vi "Clear.vi"(8 "error in (no error)":errorcluster, 11 "Engine Simulation Session":refnum<class "Engine Simulation Session.lvclass">) -> (0 "error out":errorcluster)   [LabVIEW 2013, in "Engine Simulation Session.lvclass"]
uses:
  Engine Simulation Session.lvclass
  Engine Simulation Session.lvclass/Engine Simulation Session.ctl
  <vilib>/FPGAPlugInAG/Dynamic/niLvFpga_Close_Dynamic.vi
  <vilib>/rvi/interface/nirviCloseFPGA/nirviCloseFPGA.xnode
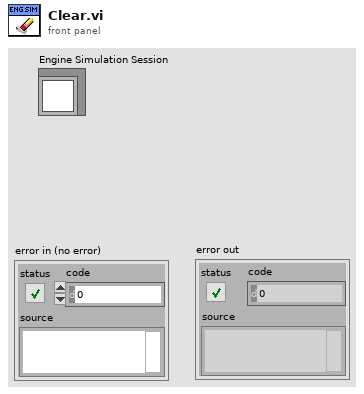
[diagram p1: front panel]
types:
  T1 = typedef "Engine Simulation Session.lvclass/session class private data.ctl" = cluster{"running":bool, "fpga reference":refnum<k20>, "bitfile":path}
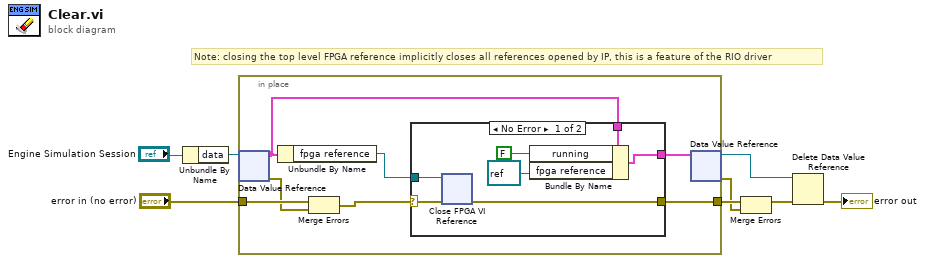
[diagram p0: block diagram]
diagram:
  # "Note: closing the top level FPGA reference implicitly closes all references opened by IP, this is a feature of the RIO driver"
  n1 = Unbundle By Name("Engine Simulation Session") -> ("data"=w7:refnum<data-value>)
  n2 = in-place {
    in-place-border: "error in (no error)" -> [w13]
    in-place-border: [w11] -> w5
    n3 = in-place-dvr #1(w7) -> (w15:T1, w10:errorcluster)
    n4 = Unbundle By Name(w15) -> ("fpga reference"=w12:refnum<k20>)
    n5 = Merge Errors(w13, w10) -> (w9:errorcluster)
    n6 = case shown="No Error" w9 {
      selector: w9 -> [w16 w23]
      tunnel: w15 -> [w22 w24]
      tunnel: [w20 w24] -> w14
      tunnel: w12 -> [w19 _]
      tunnel: [w18 w23] -> w11
      frame No Error {
        n7 = xnode "Close FPGA VI Reference"("FPGA VI Reference In"=w19, "error in"=w16) -> ("error out"=w18:errorcluster)
        n8 = Bundle By Name(cluster=w22, "running"=FALSE, "fpga reference"=refnum<k20> refnum) -> (w20:T1)
      }
      frame Error {
      }
    }
    n9 = in-place-dvr #1(w14) -> (w1:refnum<data-value>, w4:errorcluster)
  }
  n10 = Merge Errors(w5, w4) -> (w3:errorcluster)
  n11 = Delete Data Value Reference(data value reference=w1, error in=w3) -> (error out=→"error out":errorcluster)  [unwired: 1 out]
